vi "set_cold_juntion_compensation.vi"(8 "error in (no error)":errorcluster, 10 "Enable":bool, 11 "Modbus Master in":refnum<class "Modbus Master.lvclass">) -> (0 "error out":errorcluster, 3 "Modbus Master out":refnum<class "Modbus Master.lvclass">)   [LabVIEW 2018]
uses:
  <vilib>/NI/Modbus Library/API/Master/Modbus Master.lvclass
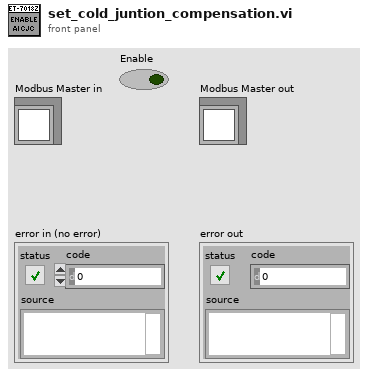
[diagram p1: front panel]
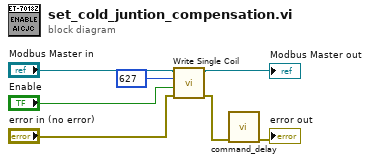
[diagram p0: block diagram]
diagram:
  n1 = call-dynamic "Write Single Coil.vi"("error in"="error in (no error)", "coil to write"="Enable", "address"=u16 627 ("starting address"), "Modbus master in"="Modbus Master in") -> ("error out"=w1:errorcluster, "Modbus master out"=→"Modbus Master out":refnum<class "Modbus Master.lvclass">)  [unwired: 6 in]
  n2 = call "command_delay.vi"("error in (no error)"=w1) -> ("error out"=→"error out":errorcluster)  [unwired: 10 in]
